vi "Main_16a.vi"() -> ()   [LabVIEW 2023]
panel:
  out "Answer":i32
  in  "Puzzle":string="Valve DB has flow rate=0; tunnels lead to valves AC, UN\nValve LC has flow rate=6; tunnels lead to valves UV, CM, RD, IM, YQ\nValve SU has flow rate=0; tunnels lead to valves OH, BX\nValve JS has flow rate=0; tunnels lead to valves GR, RW\nValve BX has flow rate=18; tunnels lead to valves PA, SU\nValve WI has flow rate=0; tunnels lead to valves GR, JI\nValve YQ has flow rate=0; tunnels lead to valves LC, SB\nValve HX has flow rate=10; tunnels lead to valves VR, GZ, ID\nValve RI has flow rate=0; tunnels lead to valves HF, UV\nValve JQ has flow rate=0; tunnels lead to valves AA, IF\nValve RK has flow rate=0; tunnels lead to valves AA, CM\nValve AC has flow rate=0; tunnels lead to valves DB, HF\nValve JI has flow rate=12; tunnels lead to valves WI, YH, ND, ID\nValve DF has flow rate=0; tunnels lead to valves JW, AA\nValve PA has flow rate=0; tunnels lead to valves BX, RB\nValve OU has flow rate=0; tunnels lead to valves OH, XM\nValve YO has flow rate=0; tunnels lead to valves OK, HF\nValve YY has flow rate=0; tunnels lead to valves UN, MC\nValve OJ has flow rate=0; tunnels lead to valves SC, GR\nValve VR has flow rate=0; tunnels lead to valves IR, HX\nValve EY has flow rate=0; tunnels lead to valves HR, OK\nValve LE has flow rate=0; tunnels lead to valves GV, GZ\nValve HF has flow rate=14; tunnels lead to valves DS, YO, AC, RI, WP\nValve OM has flow rate=0; tunnels lead to valves DS, GV\nValve JW has flow rate=0; tunnels lead to valves UN, DF\nValve OK has flow rate=9; tunnels lead to valves IF, EY, OV, YO, WM\nValve RB has flow rate=0; tunnels lead to valves PA, XM\nValve HR has flow rate=0; tunnels lead to valves EY, CQ\nValve YM has flow rate=0; tunnels lead to valves GB, NB\nValve UN has flow rate=5; tunnels lead to valves RD, DB, JW, YY, WC\nValve SO has flow rate=0; tunnels lead to valves AA, RH\nValve RW has flow rate=0; tunnels lead to valves JS, GV\nValve IF has flow rate=0; tunnels lead to valves OK, JQ\nValve WP has flow rate=0; tunnels lead to valves HF, CQ\nValve YK has flow rate=0; tunnels lead to valves MO, GV\nValve MQ has flow rate=0; tunnels lead to valves AA, HI\nValve RH has flow rate=0; tunnels lead to valves SO, GB\nValve GB has flow rate=7; tunnels lead to valves YM, RH, PU\nValve XM has flow rate=16; tunnels lead to valves OU, ND, NB, RB\nValve RD has flow rate=0; tunnels lead to valves UN, LC\nValve HI has flow rate=0; tunnels lead to valves MQ, GR\nValve OH has flow rate=19; tunnels lead to valves OU, SU\nValve DS has flow rate=0; tunnels lead to valves OM, HF\nValve GV has flow rate=24; tunnels lead to valves RW, MC, YK, OM, LE\nValve AA has flow rate=0; tunnels lead to valves SO, DF, RK, MQ, JQ\nValve CQ has flow rate=17; tunnels lead to valves SB, MO, WP, SC, HR\nValve UV has flow rate=0; tunnels lead to valves LC, RI\nValve OV has flow rate=0; tunnels lead to valves OK, WC\nValve CM has flow rate=0; tunnels lead to valves RK, LC\nValve YH has flow rate=0; tunnels lead to valves NW, JI\nValve GZ has flow rate=0; tunnels lead to valves LE, HX\nValve WC has flow rate=0; tunnels lead to valves UN, OV\nValve ID has flow rate=0; tunnels lead to valves JI, HX\nValve SC has flow rate=0; tunnels lead to valves OJ, CQ\nValve GR has flow rate=11; tunnels lead to valves OJ, WI, HI, PU, JS\nValve IM has flow rate=0; tunnels lead to valves LC, WM\nValve NB has flow rate=0; tunnels lead to valves YM, XM\nValve TS has flow rate=20; tunnel leads to valve NW\nValve SB has flow rate=0; tunnels lead to valves CQ, YQ\nValve MC has flow rate=0; tunnels lead to valves GV, YY\nValve ND has flow rate=0; tunnels lead to valves JI, XM\nValve MO has flow rate=0; tunnels lead to valves CQ, YK\nValve PU has flow rate=0; tunnels lead to valves GB, GR\nValve IR has flow rate=13; tunnel leads to valve VR\nValve NW has flow rate=0; tunnels lead to valves YH, TS\nValve WM has flow rate=0; tunnels lead to valves IM, OK"
  in  "Example":string="Valve AA has flow rate=0; tunnels lead to valves DD, II, BB\nValve BB has flow rate=13; tunnels lead to valves CC, AA\nValve CC has flow rate=2; tunnels lead to valves DD, BB\nValve DD has flow rate=20; tunnels lead to valves CC, AA, EE\nValve EE has flow rate=3; tunnels lead to valves FF, DD\nValve FF has flow rate=0; tunnels lead to valves EE, GG\nValve GG has flow rate=0; tunnels lead to valves FF, HH\nValve HH has flow rate=22; tunnel leads to valve GG\nValve II has flow rate=0; tunnels lead to valves AA, JJ\nValve JJ has flow rate=21; tunnel leads to valve II"
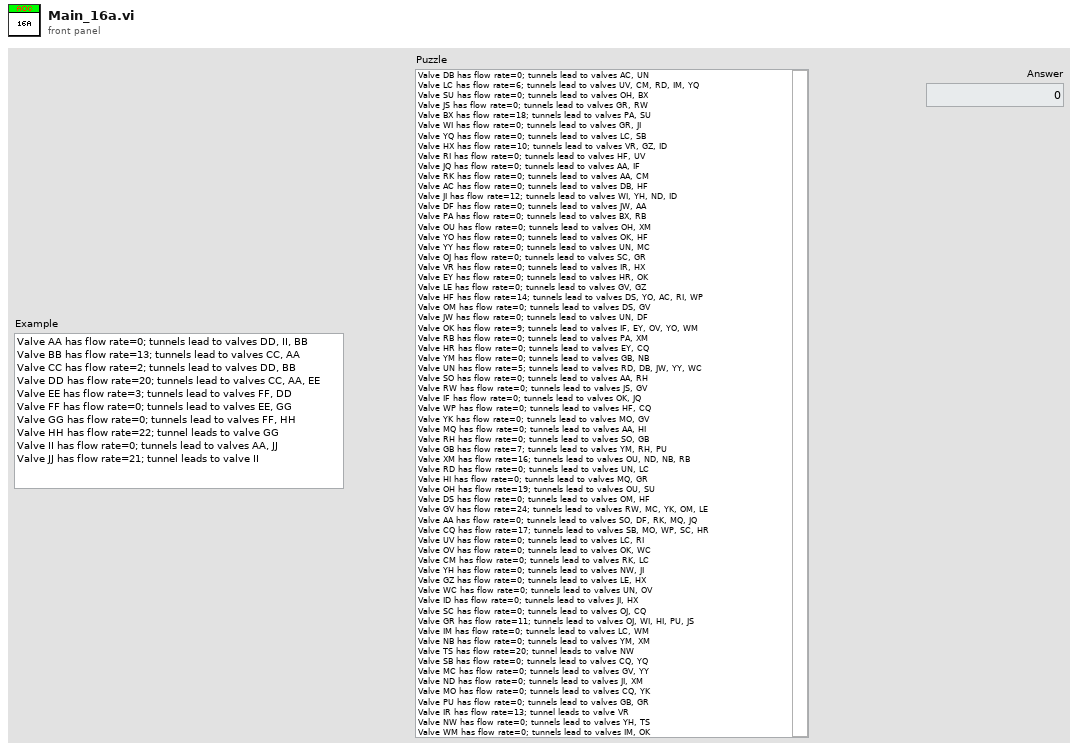
[diagram p1: front panel]
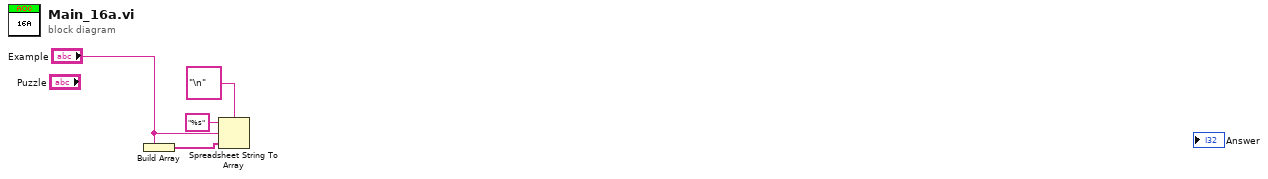
[diagram p0: block diagram]
diagram:
  n1 = Build Array("Example") -> (w4:string[])
  n2 = Spreadsheet String To Array(delimiter (Tab)="\n", format string="%s", spreadsheet string="Example", array type (2D Dbl)=w4) -> ()  [unwired: 1 out]
